vi "libssh2_sftp_fstat_ex.vi"(8 "error in (no error)":errorcluster, 9 "set":bool, 10 "attributes in":T1, 11 "sftp handle":T2) -> (0 "error out":errorcluster, 2 "attributes out":T1)   [LabVIEW 2017, in "libssh2.lvlib"]
doc: "Get or set the attributes of a file handle."
uses:
  libssh2.lvlib
  SFTP Handle Refnum.ctl
  libssh2_sftp_attributes.ctl
  Acquire SFTP.vi
  Release SFTP.vi
  Acquire Session.vi
  Release Session.vi
  Not An SFTP Handle Refnum.vi
  <vilib>/Utility/error.llb/Error Cluster From Error Code.vi
  Global Settings.vi
  Read SFTP Handle Refnum.vi
  Read SFTP Refnum.vi
  Read Session Refnum.vi
  <vilib>/Utility/semaphor.llb/Acquire Semaphore.vi
  <vilib>/Utility/semaphor.llb/Release Semaphore.vi
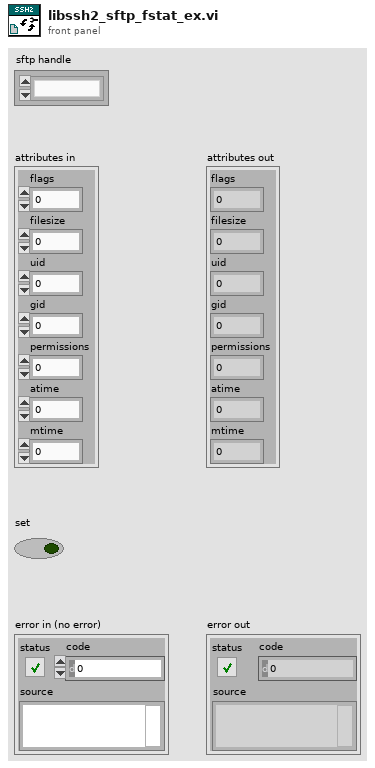
[diagram p1: front panel]
types:
  T1 = typedef "libssh2.lvlib/libssh2_sftp_attributes.ctl" = cluster{"flags":u32, "filesize":u64, "uid":u32, "gid":u32, "permissions":u32, "atime":u32, "mtime":u32}
  T2 = typedef "libssh2.lvlib/SFTP Handle Refnum.ctl" = refnum<k1>
  T3 = cluster{"flags":u32, "<padding1>":u32, "filesize":u64, "uid":u32, "gid":u32, "permissions":u32, "atime":u32, "mtime":u32, "<padding2>":u32}
  T4 = cluster{"flags":u32, "<padding1>":u32, "filesize":u64, "uid":u32, "<padding2>":u32, "gid":u32, "<padding3>":u32, "permissions":u32, "<padding4>":u32, "atime":u32, "<padding5>":u32, "mtime":u32, "<padding6>":u32}
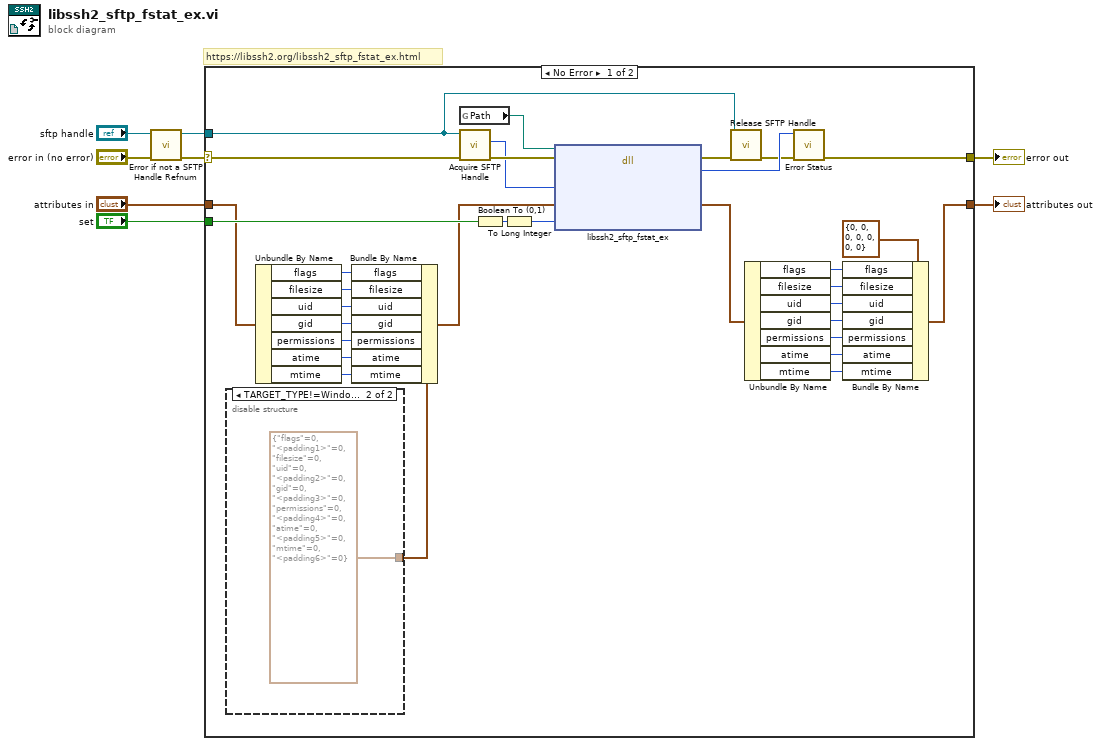
[diagram p0: block diagram]
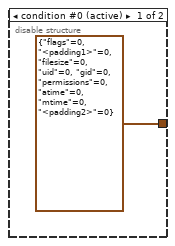
[diagram p2: hidden frame]
diagram:
  # "https://libssh2.org/libssh2_sftp_fstat_ex.html"
  n1 = call "Error if not a SFTP Handle Refnum.vi"("error in (no error)"="error in (no error)", "sftp handle"="sftp handle") -> ("error out"=w7:errorcluster, "sftp handle out"=w6:T2)  [unwired: 8 in]
  n2 = case shown="No Error" w7 {
    selector: w7 -> [w40 w44]
    tunnel: w6 -> [w35 _]
    tunnel: [w39 w44] -> w5
    tunnel: "set" -> [w38 _]
    tunnel: "attributes in" -> [w37 w43]
    tunnel: [w36 w43] -> w1
    frame No Error {
      n3 = disable-structure shown="TARGET_TYPE!=Windows&&TARGET_BITNESS==64" {
        disable-tunnel: [T3 {"flags"=0, "<padding1>"=0, "filesize"=0, "uid"=0, "gid"=0, "permissions"=0, "atime"=0, "mtime"=0, "<padding2>"=0} ("attrs") T4 {"flags"=0, "<padding1>"=0, "filesize"=0, "uid"=0, "<padding2>"=0, "gid"=0, "<padding3>"=0, "permissions"=0, "<padding4>"=0, "atime"=0, "<padding5>"=0, "mtime"=0, "<padding6>"=0} ("attrs")] -> w9
        frame condition #0 (active) {
        }
        frame condition #1 {
        }
      }
      n4 = Unbundle By Name(w37) -> ("flags"=w17:u32, "filesize"=w16:u64, "uid"=w15:u32, "gid"=w14:u32, "permissions"=w13:u32, "atime"=w12:u32, "mtime"=w11:u32)
      n5 = Bundle By Name(cluster=w9, "flags"=w17, "filesize"=w16, "uid"=w15, "gid"=w14, "permissions"=w13, "atime"=w12, "mtime"=w11) -> (w27:T3)
      n6 = global read "Global Settings.vi" "Path"() -> (w34:path)
      n7 = call "Acquire SFTP Handle.vi"("error in (no error)"=w40, "sftp handle"=w35) -> ("error out"=w33:errorcluster, "LIBSSH2_SFTP_HANDLE*"=w32:u64)  [unwired: 8 in]
      n8 = Boolean To (0,1)(Boolean=w38) -> (0, 1=w29:i16)
      n9 = To Long Integer(number=w29) -> (32bit integer=w28:i32)
      n10 = dll-call lib="?" fn="libssh2_sftp_fstat_ex"(path in=w34, error in=w33, "handle"=w32, "attrs"=w27, "setstat"=w28) -> (error out=w31:errorcluster, "return value"=w30:i32, "attrs"=w26:T3)  [unwired: 3 in, 1 out]
      n11 = call "Release SFTP Handle.vi"("error in (no error)"=w31, "sftp handle"=w35) -> ("error out"=w10:errorcluster)  [unwired: 9 in]
      n12 = Unbundle By Name(w26) -> ("flags"=w24:u32, "filesize"=w23:u64, "uid"=w22:u32, "gid"=w21:u32, "permissions"=w20:u32, "atime"=w19:u32, "mtime"=w18:u32)
      n13 = call "Error Status.vi"("error in (no error)"=w10, "return value"=w30) -> ("error out"=w39:errorcluster)  [unwired: 8 in, 1 out]
      n14 = Bundle By Name(cluster=T1 {"flags"=0, "filesize"=0, "uid"=0, "gid"=0, "permissions"=0, "atime"=0, "mtime"=0} ("attributes"), "flags"=w24, "filesize"=w23, "uid"=w22, "gid"=w21, "permissions"=w20, "atime"=w19, "mtime"=w18) -> (w36:T1)
    }
    frame Error {
    }
  }
  "error out" <- w5
  "attributes out" <- w1
